vi "VI-Get Private Data Cluster.vi"(0 "LabVIEW Class In":refnum<vi>, 11 "error in (no error)":errorcluster) -> (4 "LabVIEW Class Out":refnum<vi>, 6 "private data VI":refnum<vi>, 8 "private data cluster":refnum<vi>, 10 "serialized cluster":refnum<vi>, 15 "error out":errorcluster)   [LabVIEW 2020]
uses:
  <vilib>/Utility/traverseref.llb/TRef TravTarget.ctl
  <vilib>/Utility/traverseref.llb/VI Scripting - Traverse.lvlib
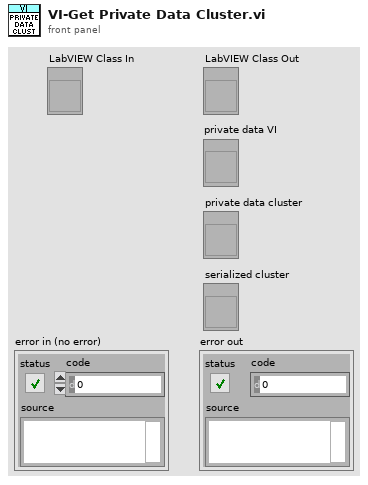
[diagram p1: front panel]
types:
  T1 = typedef "TRef TravTarget.ctl" = enum16{"FP", "BD", "Other"}
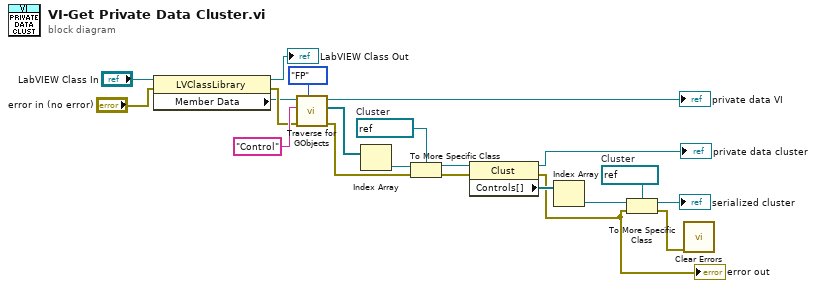
[diagram p0: block diagram]
diagram:
  w8 = refnum<vi> refnum  # Cluster
  w21 = refnum<vi> refnum  # Cluster
  n1 = property class="LVClassLibrary"(reference="LabVIEW Class In", error in="error in (no error)") -> (reference out=→"LabVIEW Class Out":refnum<vi>, error out=w13:errorcluster, "Member Data"=w12:refnum<vi>)
  n2 = call <vilib>:"Traverse for GObjects.vi"("Traverse Target"=TRef_TravTarget."FP", "error in (no error)"=w13, "Class Name"="Control", "VI Refnum"=w12) -> ("error out"=w16:errorcluster, "References"=w18:refnum<vi>[], "dup VI Refnum"=→"private data VI":refnum<vi>)  [unwired: 4 in, 1 out]
  n3 = Index Array(array=w18) -> (element=w17:refnum<vi>)  [unwired: 1 in]
  n4 = To More Specific Class(target class=w21, reference=w17, error in=w16) -> (specific class reference=w6:refnum<vi>, error out=w7:errorcluster)
  n5 = property class="Clust"(reference=w6, error in=w7) -> (reference out=→"private data cluster":refnum<vi>, error out=w2:errorcluster, "Controls[]"=w10:refnum<vi>[])
  "error out" <- w2
  n6 = Index Array(array=w10) -> (element=w9:refnum<vi>)  [unwired: 1 in]
  n7 = To More Specific Class(target class=w8, reference=w9, error in=w2) -> (specific class reference=→"serialized cluster":refnum<vi>, error out=w1:errorcluster)
  n8 = call <vilib>:"Clear Errors.vi"("error in (no error)"=w1) -> ()  [unwired: 5 in, 2 out]
